vi "Test_WriteInitialList_RetrieveList.vi"(8 "error in (no error)":errorcluster, 11 "TestCase in":refnum<class "TestStringList.lvclass">) -> (0 "error out":errorcluster, 3 "TestCase out":refnum<class "TestStringList.lvclass">)   [LabVIEW 2015, in "TestStringList.lvclass"]
uses:
  TestStringList.lvclass
  <vilib>/addons/_JKI Toolkits/VI Tester/TestCase.llb/TestCase.lvclass
  StringList.lvclass
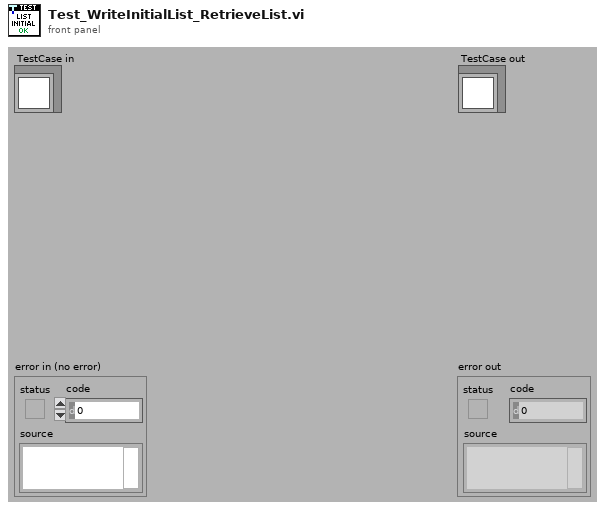
[diagram p1: front panel]
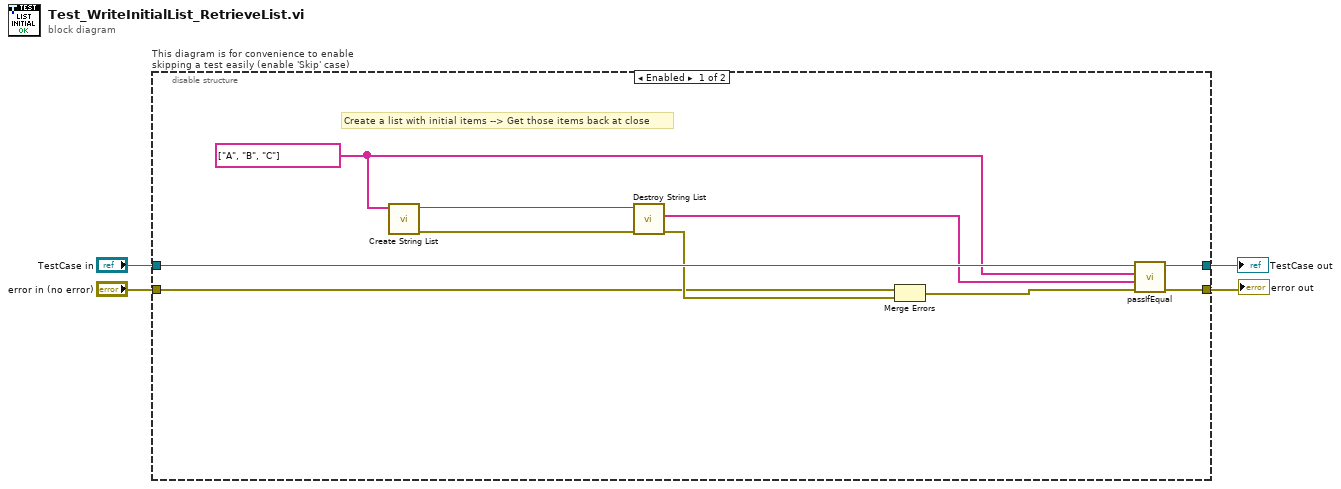
[diagram p0: block diagram]
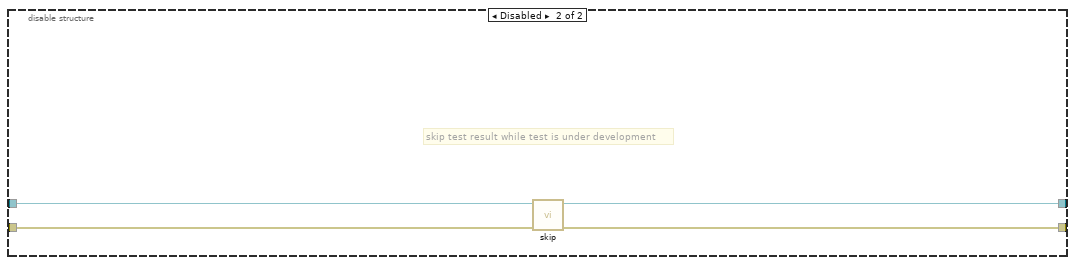
[diagram p2: hidden frame]
diagram:
  n1 = disable-structure "This diagram is for convenience to enable skipping a test easily (enable 'Skip' case)" shown="Enabled" {
    disable-tunnel: "TestCase in" -> [w14 w18]
    disable-tunnel: [w13 w16] -> w1
    disable-tunnel: [w12 w17] -> w3
    disable-tunnel: "error in (no error)" -> [w9 w15]
    frame Enabled {
      w6 = string[] ["A", "B", "C"] ("Initial Strings (empty list)")
      # "Create a list with initial items --> Get those items back at close"
      n2 = call "Create String List.vi"("Initial Strings (empty list)"=w6) -> ("error out"=w7:errorcluster, "StringList Reference"=w8:refnum<data-value>)  [unwired: 9 in]
      n3 = call "Destroy String List.vi"("error in (no error)"=w7, "StringList Reference"=w8) -> ("error out"=w10:errorcluster, "Final Items"=w5:string[])  [unwired: 8 in]
      n4 = Merge Errors(w9, w10) -> (w11:errorcluster)
      n5 = call-dynamic "passIfEqual.vi"("error in (no error)"=w11, "y"=w5, "x"=w6, "TestCase in"=w14) -> ("error out"=w12:errorcluster, "TestCase out"=w13:refnum<class "TestStringList.lvclass">)  [unwired: 6 in]
    }
    frame Disabled {
      # "skip test result while test is under development"
      n6 = call <vilib>:"skip.vi"("error in (no error)"=w15, "TestCase in"=w18) -> ("error out"=w17:errorcluster, "TestCase out"=w16:refnum<class "TestStringList.lvclass">)  [unwired: 8 in]
    }
  }
  "error out" <- w3
  "TestCase out" <- w1
